vi "Do[Core].vi"(0 "ControlAction in":refnum<class "ControlActionBase.lvclass">, 5 "Ctl Refnum in":refnum<vi>, 11 "error in (no error)":errorcluster) -> (4 "ControlAction out":refnum<class "ControlActionBase.lvclass">, 6 "Ctl Refnum out":refnum<vi>, 15 "error out":errorcluster)   [LabVIEW 2016, in "ControlActionBase.lvclass"]
uses:
  ControlActionBase.lvclass
  ControlActionBase.lvclass/ControlActionBase.ctl
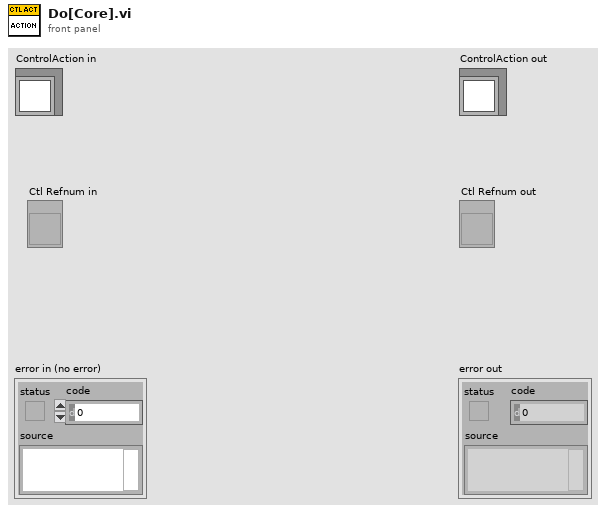
[diagram p1: front panel]
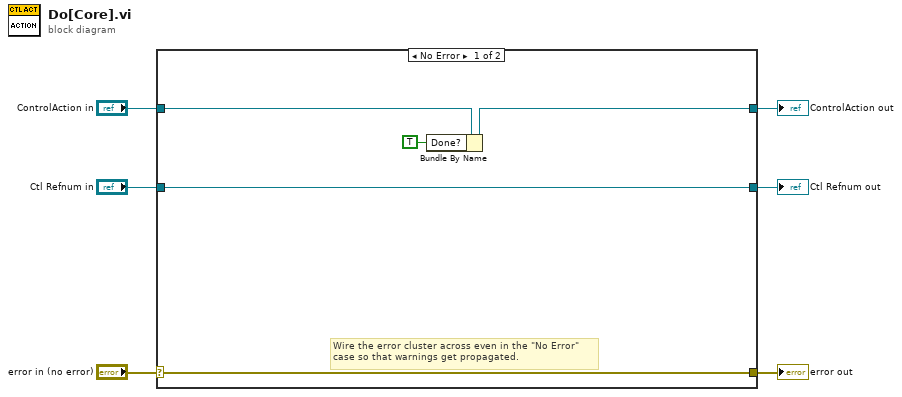
[diagram p0: block diagram]
diagram:
  n1 = case shown="No Error" "error in (no error)" {
    selector: "error in (no error)" -> [w10 w14]
    tunnel: [w10 w14] -> w5
    tunnel: [w8 w13] -> w3
    tunnel: "ControlAction in" -> [w11 w13]
    tunnel: [w9 w12] -> w2
    tunnel: "Ctl Refnum in" -> [w9 w12]
    frame No Error {
      # "Wire the error cluster across even in the \"No Error\"\ncase so that warnings get propagated."
      n2 = Bundle By Name(cluster=w11, "Done?"=TRUE) -> (w8:refnum<class "ControlActionBase.lvclass">)
    }
    frame Error {
    }
  }
  "error out" <- w5
  "ControlAction out" <- w3
  "Ctl Refnum out" <- w2
